vi "generateFPGADataTelemetryEvent.vi"(8 "error in (no error)":errorcluster, 10 "TelemetryFPGAData":T1, 11 "UserEvents in":refnum<class "UserEvents.lvclass">) -> (0 "error out":errorcluster, 3 "UserEvents out":refnum<class "UserEvents.lvclass">)   [LabVIEW 2016, in "UserEvents.lvclass"]
uses:
  UserEvents.lvclass
  Communicator/Topics/TelemetryFPGAData.ctl
  Types/Timestamp.ctl
  UserEvents.lvclass/UserEvents.ctl
  Types/M1M3SupportTypes.lvlib
  Communicator/M1M3Communicator.lvlib
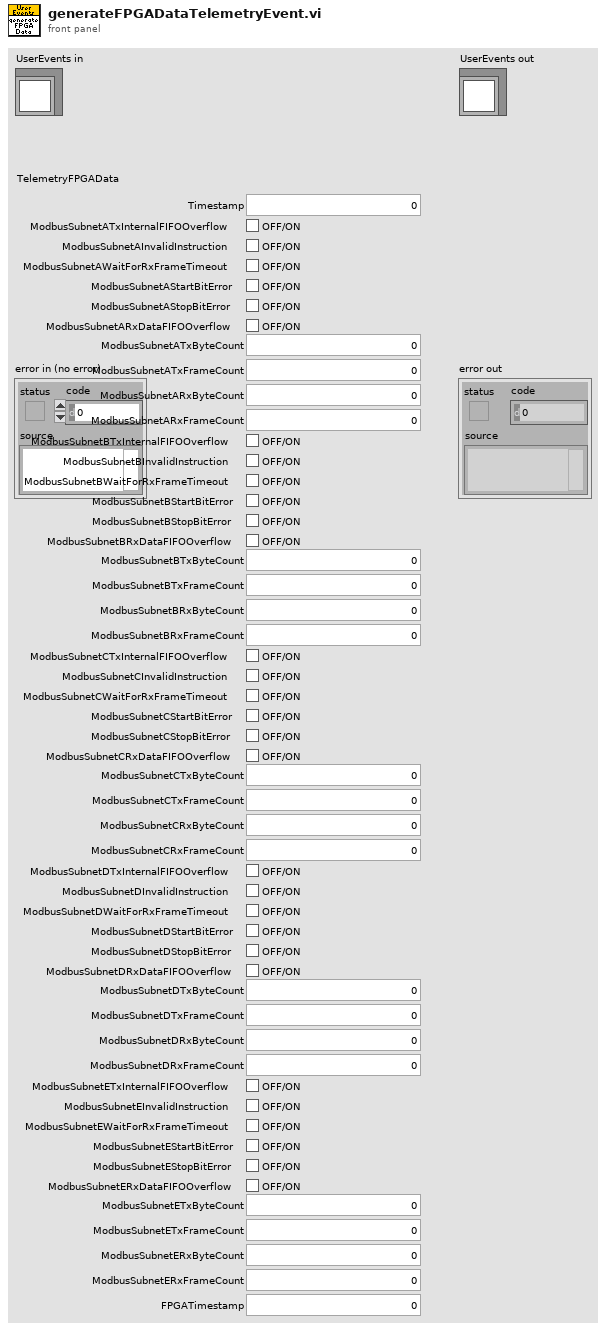
[diagram p1: front panel]
types:
  T1 = typedef "M1M3Communicator.lvlib/TelemetryFPGAData.ctl" = cluster{"Timestamp":T2, "ModbusSubnetATxInternalFIFOOverflow":bool, "ModbusSubnetAInvalidInstruction":bool, "ModbusSubnetAWaitForRxFrameTimeout":bool, "ModbusSubnetAStartBitError":bool, "ModbusSubnetAStopBitError":bool, "ModbusSubnetARxDataFIFOOverflow":bool, "ModbusSubnetATxByteCount":i32, "ModbusSubnetATxFrameCount":i32, "ModbusSubnetARxByteCount":i32, "ModbusSubnetARxFrameCount":i32, "ModbusSubnetBTxInternalFIFOOverflow":bool, "ModbusSubnetBInvalidInstruction":bool, "ModbusSubnetBWaitForRxFrameTimeout":bool, "ModbusSubnetBStartBitError":bool, "ModbusSubnetBStopBitError":bool, "ModbusSubnetBRxDataFIFOOverflow":bool, "ModbusSubnetBTxByteCount":i32, "ModbusSubnetBTxFrameCount":i32, "ModbusSubnetBRxByteCount":i32, "ModbusSubnetBRxFrameCount":i32, "ModbusSubnetCTxInternalFIFOOverflow":bool, "ModbusSubnetCInvalidInstruction":bool, "ModbusSubnetCWaitForRxFrameTimeout":bool, "ModbusSubnetCStartBitError":bool, "ModbusSubnetCStopBitError":bool, "ModbusSubnetCRxDataFIFOOverflow":bool, "ModbusSubnetCTxByteCount":i32, "ModbusSubnetCTxFrameCount":i32, "ModbusSubnetCRxByteCount":i32, "ModbusSubnetCRxFrameCount":i32, "ModbusSubnetDTxInternalFIFOOverflow":bool, "ModbusSubnetDInvalidInstruction":bool, "ModbusSubnetDWaitForRxFrameTimeout":bool, "ModbusSubnetDStartBitError":bool, "ModbusSubnetDStopBitError":bool, "ModbusSubnetDRxDataFIFOOverflow":bool, "ModbusSubnetDTxByteCount":i32, "ModbusSubnetDTxFrameCount":i32, "ModbusSubnetDRxByteCount":i32, "ModbusSubnetDRxFrameCount":i32, "ModbusSubnetETxInternalFIFOOverflow":bool, "ModbusSubnetEInvalidInstruction":bool, "ModbusSubnetEWaitForRxFrameTimeout":bool, "ModbusSubnetEStartBitError":bool, "ModbusSubnetEStopBitError":bool, "ModbusSubnetERxDataFIFOOverflow":bool, "ModbusSubnetETxByteCount":i32, "ModbusSubnetETxFrameCount":i32, "ModbusSubnetERxByteCount":i32, "ModbusSubnetERxFrameCount":i32, "FPGATimestamp":dbl}
  T2 = typedef "M1M3SupportTypes.lvlib/Timestamp.ctl" = dbl
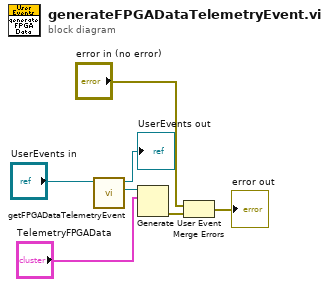
[diagram p0: block diagram]
diagram:
  n1 = call "getFPGADataTelemetryEvent.vi"("UserEvents in"="UserEvents in") -> ("FPGADataTelemetryEvent"=w7:refnum<user-event>, "UserEvents out"=→"UserEvents out":refnum<class "UserEvents.lvclass">)  [unwired: 9 in]
  n2 = Generate User Event(user event=w7, event data cluster="TelemetryFPGAData") -> (error out=w3:errorcluster)  [unwired: 2 in, 1 out]
  n3 = Merge Errors("error in (no error)", w3) -> (→"error out":errorcluster)
